vi "subGenerateModulationSchemes.vi"(11 "error in (no error)":errorcluster) -> (4 "Modulation Schemes":cluster{"Symbol Map":cdb[], "bits/symbol":i32}[](array[cluster]), 15 "error out":errorcluster)   [LabVIEW 2011]
uses:
  <vilib>/addons/Modulation/niDMT.lvlib
  <vilib>/Analysis/NI_AALBase.lvlib
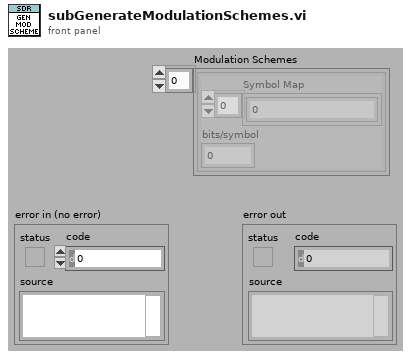
[diagram p1: front panel]
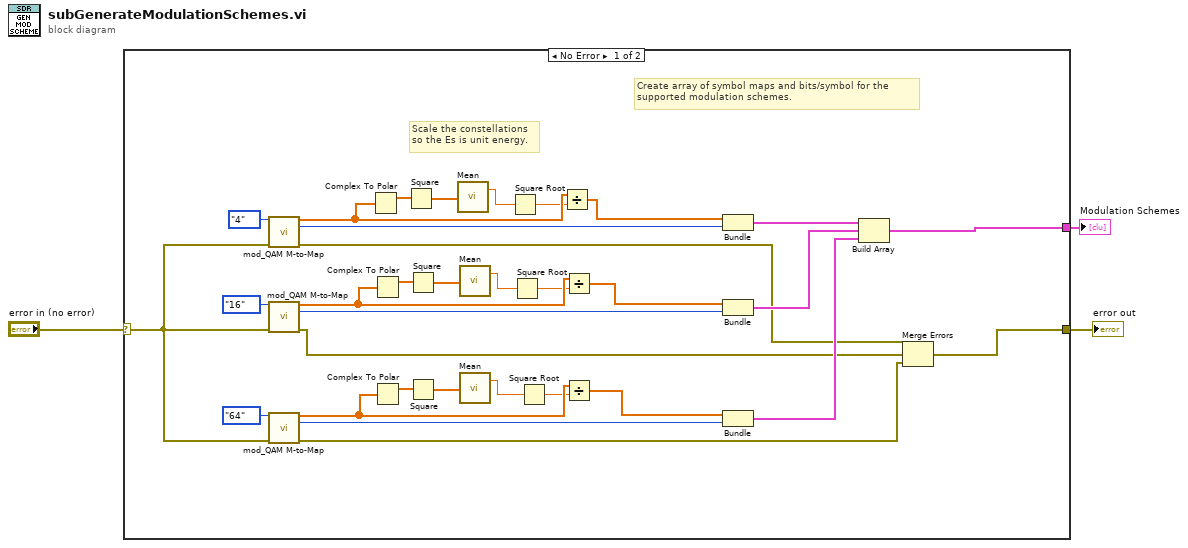
[diagram p0: block diagram]
diagram:
  n1 = case shown="No Error" "error in (no error)" {
    selector: "error in (no error)" -> [w30 w37]
    tunnel: [w22 w37] -> w2
    tunnel: [w23 _] -> w1
    frame No Error {
      # "Scale the constellations \nso the Es is unit energy."
      # "Create array of symbol maps and bits/symbol for the \nsupported modulation schemes."
      n2 = call <vilib>:"mod_QAM M-to-Map.vi"("M selection"=enum16{"4", "8", "16", "32", "64", "128", "256"}."4", "error in (no error)"=w30) -> ("Symbol Map"=w18:cdb[], "bits/symbol"=w35:i32, "error out"=w26:errorcluster)  [unwired: 11 out]
      n3 = call <vilib>:"mod_QAM M-to-Map.vi"("M selection"=enum16{"4", "8", "16", "32", "64", "128", "256"}."16", "error in (no error)"=w30) -> ("Symbol Map"=w14:cdb[], "bits/symbol"=w33:i32, "error out"=w25:errorcluster)  [unwired: 11 out]
      n4 = call <vilib>:"mod_QAM M-to-Map.vi"("M selection"=enum16{"4", "8", "16", "32", "64", "128", "256"}."64", "error in (no error)"=w30) -> ("Symbol Map"=w11:cdb[], "bits/symbol"=w31:i32, "error out"=w24:errorcluster)  [unwired: 11 out]
      n5 = Complex To Polar(r * e^(i*theta)=w18) -> (r=w21:dbl[])  [unwired: 1 out]
      n6 = Complex To Polar(r * e^(i*theta)=w14) -> (r=w15:dbl[])  [unwired: 1 out]
      n7 = Complex To Polar(r * e^(i*theta)=w11) -> (r=w13:dbl[])  [unwired: 1 out]
      n8 = Square(x=w21) -> (x^2=w20:dbl[])
      n9 = Square(x=w15) -> (x^2=w16:dbl[])
      n10 = Square(x=w13) -> (x^2=w12:dbl[])
      n11 = call <vilib>:"Mean.vi"("X"=w20) -> ("mean"=w19:dbl)  [unwired: 1 out]
      n12 = call <vilib>:"Mean.vi"("X"=w16) -> ("mean"=w17:dbl)  [unwired: 1 out]
      n13 = call <vilib>:"Mean.vi"("X"=w12) -> ("mean"=w8:dbl)  [unwired: 1 out]
      n14 = Square Root(x=w19) -> (sqrt(x)=w6:dbl)
      n15 = Square Root(x=w17) -> (sqrt(x)=w7:dbl)
      n16 = Square Root(x=w8) -> (sqrt(x)=w9:dbl)
      n17 = Divide(x=w18, y=w6) -> (x/y=w4:cdb[])
      n18 = Divide(x=w14, y=w7) -> (x/y=w5:cdb[])
      n19 = Divide(x=w11, y=w9) -> (x/y=w10:cdb[])
      n20 = Bundle(w4, "bits/symbol"=w35) -> (w29:cluster{cdb[], "bits/symbol":i32})  [unwired: 1 out]
      n21 = Bundle(w5, "bits/symbol"=w33) -> (w28:cluster{cdb[], "bits/symbol":i32})  [unwired: 1 out]
      n22 = Bundle(w10, "bits/symbol"=w31) -> (w27:cluster{cdb[], "bits/symbol":i32})  [unwired: 1 out]
      n23 = Build Array(w29, w28, w27) -> (w23:cluster{cdb[], "bits/symbol":i32}[])
      n24 = Merge Errors(w26, w25, w24) -> (w22:errorcluster)
    }
    frame Error {
    }
  }
  "error out" <- w2
  "Modulation Schemes" <- w1
